vi "判斷回原點.vi"(1 "¬}y":i32, 2 "¬}x":dbl, 3 "¤Hy":i32, 4 "¤Hx":dbl) -> (0 "x .and. y?":bool)   [LabVIEW 2014]
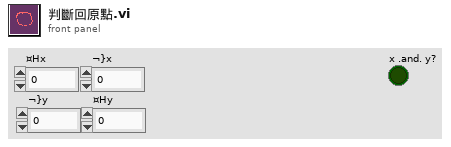
[diagram p1: front panel]
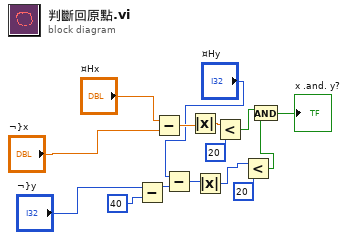
[diagram p0: block diagram]
diagram:
  n1 = Subtract(x="¬}y", y=40) -> (x-y=w12:i32)
  n2 = Subtract(x="¤Hx", y="¬}x") -> (x-y=w15:dbl)
  n3 = Subtract(x="¤Hy", y=w12) -> (x-y=w9:i32)
  n4 = Absolute Value(x=w15) -> (abs(x)=w13:dbl)
  n5 = Absolute Value(x=w9) -> (abs(x)=w7:i32)
  n6 = Less?(x=w13, y=20) -> (x < y?=w14:bool)
  n7 = Less?(x=w7, y=20) -> (x < y?=w6:bool)
  n8 = And(x=w14, y=w6) -> (x .and. y?=→"x .and. y?":bool)
